vi "Create Channel Arbitrary Waveform [ACH].vi"(8 "error in (no error)":errorcluster, 9 "waveform data array (empty)":dbl[](array[numeric]) format="%.3f", 10 "Channel Name (\"\")":string="CHANNEL1" caption="channel name (\"CHANNEL1\")", 11 "CS++Fgen in":refnum<class "CS++Fgen.lvclass">) -> (0 "error out":errorcluster, 2 "waveform handle":i32, 3 "CS++Fgen out":refnum<class "CS++Fgen.lvclass">)   [LabVIEW 2013, in "CS++Fgen.lvlib" / "CS++Fgen.lvclass"]
doc: "This VI creates a channel-specific arbitrary waveform and returns a handle that identifies that waveform. You pass this handle to the IviFgen Configure Arbitrary Waveform [ARB] VI to produce that waveform. You also use the handles this VI returns to specify a sequence of arbitrary waveforms with the IviFgen Create Arbitrary Sequence [SEQ] VI.\n\nIf the instrument does not support channel-based arbitrary waveform creation, use the IviFgen Create Arbitrary Waveform VI.\n\nUse the following VIs to create a channel-specific arbitrary waveform if you want to pass data in 16-bit or 32-bit binary:\n- IviFgen Create Channel Arbitrary Waveform Int16 [AB] VI \n- IviFgen Create Channel Arbitrary Waveform Int32 [AB] VI\n\nNote:\n\n(1) This VI is part of the IviFgenArbChannelWfm [ACH] extension group."
uses:
  CS++Fgen.lvclass
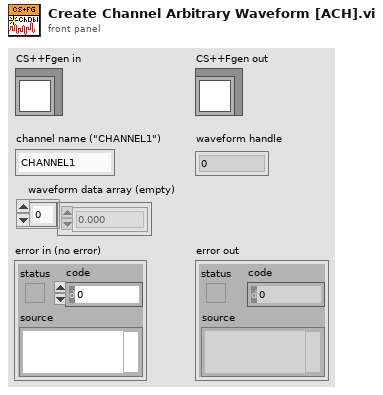
[diagram p1: front panel]
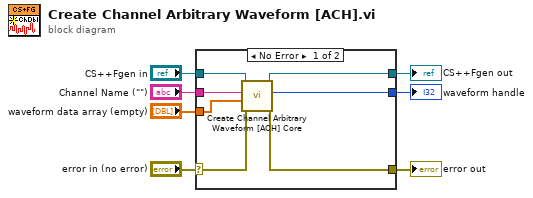
[diagram p0: block diagram]
diagram:
  n1 = case shown="No Error" "error in (no error)" {
    selector: "error in (no error)" -> [w12 w16]
    tunnel: [w11 w16] -> w6
    tunnel: [w13 w15] -> w4
    tunnel: "CS++Fgen in" -> [w14 w15]
    tunnel: "waveform data array (empty)" -> [w8 _]
    tunnel: "Channel Name (\"\")" -> [w9 _]
    tunnel: [w10 _] -> w1
    frame No Error {
      n2 = call-dynamic "Create Channel Arbitrary Waveform [ACH] Core.vi"("error in (no error)"=w12, "waveform data array (empty)"=w8, "Channel Name (\"\")"=w9, "CS++Fgen in"=w14) -> ("error out"=w11:errorcluster, "waveform handle"=w10:i32, "CS++Fgen out"=w13:refnum<class "CS++Fgen.lvclass">)  [unwired: 5 in]
    }
    frame Error {
    }
  }
  "error out" <- w6
  "CS++Fgen out" <- w4
  "waveform handle" <- w1
